vi "Hide Residuals.vi"(8 "error in (no error)":errorcluster, 10 "Residuals":bool, 11 "WaveformGraph in":refnum<vi>) -> (0 "error out":errorcluster, 3 "WaveformGraph out":refnum<vi>)   [LabVIEW 2013, in "main.lvlib"]
uses:
  main.lvlib
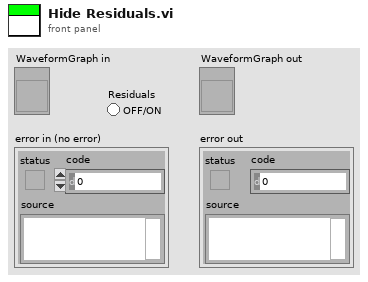
[diagram p1: front panel]
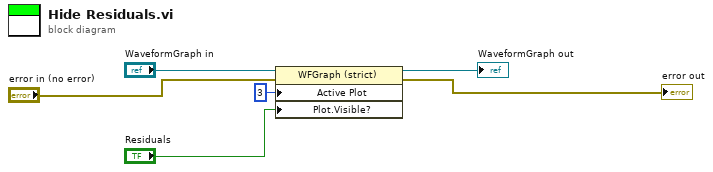
[diagram p0: block diagram]
diagram:
  n1 = property class="WFGraph (strict)"(reference="WaveformGraph in", error in="error in (no error)", "Active Plot"=u32 3, "Plot.Visible?"="Residuals") -> (reference out=→"WaveformGraph out":refnum<vi>, error out=→"error out":errorcluster)
